vi "LinkedServer.vi"() -> ()   [LabVIEW 2012]
uses:
  <vilib>/addons/database/Auxilliary.llb/DB Tools Cursor Type.ctl
  <vilib>/addons/database/Connection.llb/DB Tools Open Connec (Path).vi
  <vilib>/addons/database/Connection.llb/Conn Execute.vi
  <vilib>/addons/database/Recordset.llb/Rec Fetch Recordset Data (R).vi
  <vilib>/addons/database/Recordset.llb/Rec Destroy - Connection.vi
  <vilib>/addons/database/NI_Database_API.lvlib
panel:
  out "recordset data":variant[][](array[variant])
  out "error out":errorcluster
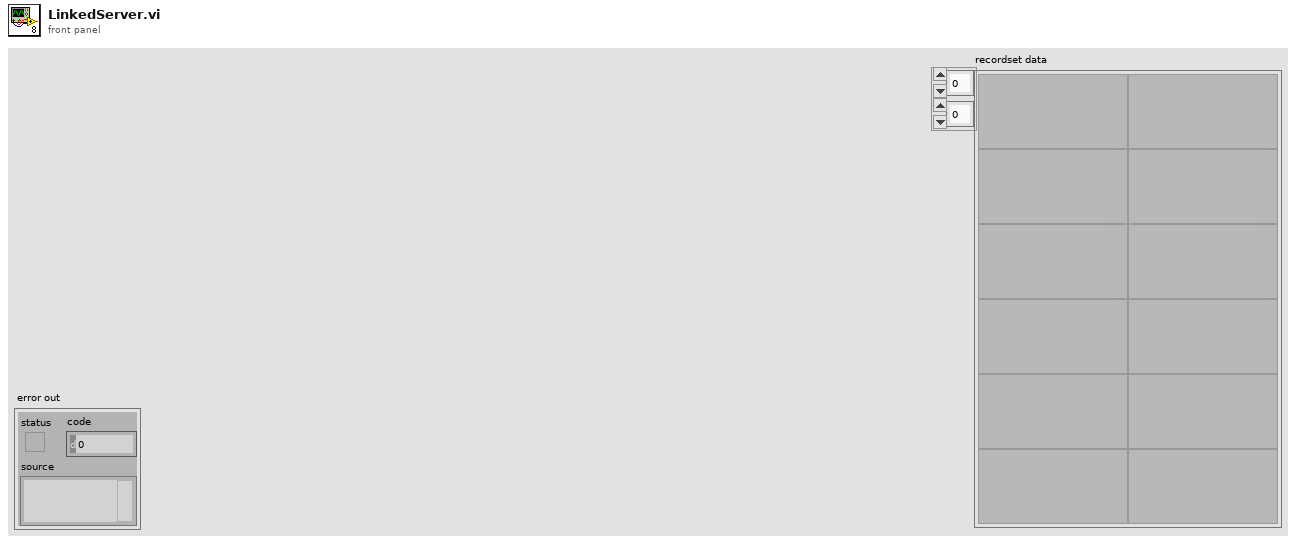
[diagram p1: front panel]
types:
  T1 = typedef "NI_Database_API.lvlib/DB Tools Cursor Type.ctl" = enum16{"forward-only", "keyset", "dynamic", "static"}
  T2 = typedef "NI_Database_API.lvlib/Conn ObjectReference.ctl" = refnum<k1>
  T3 = typedef "NI_Database_API.lvlib/Rec ObjectReference.ctl" = refnum<k1>
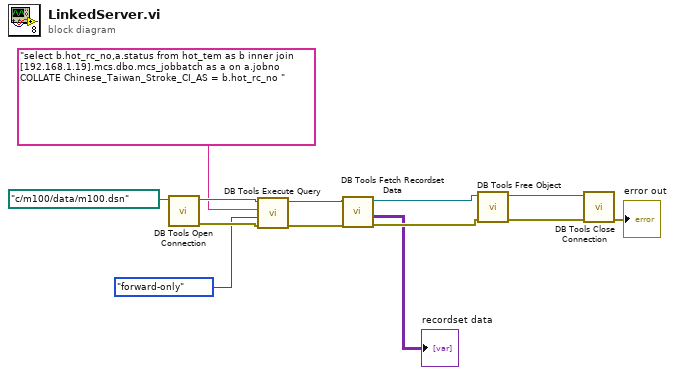
[diagram p0: block diagram]
diagram:
  n1 = call-poly <vilib>:"DB Tools Open Connection.vi"("connection information"=path "c:/m100/data/m100.dsn") -> ("error out"=w4:errorcluster, "connection reference"=w5:T2)  [unwired: 7 in]
  n2 = call-poly <vilib>:"DB Tools Execute Query.vi"("error in (no error)"=w4, "cursor type"=DB_Tools_Cursor_Type."forward-only", "SQL query"="select b.hot_rc_no,a.status from hot_tem as b inner join [192.168.1.19].mcs.dbo.mcs_jobbatch as a on a.jobno COLLATE Chinese_Taiwan_Stroke_CI_AS = b.hot_rc_no ", "connection reference"=w5) -> ("error out"=w6:errorcluster, "recordset reference"=w7:T3)  [unwired: 4 in]
  n3 = call-poly <vilib>:"DB Tools Fetch Recordset Data.vi"("error in (no error)"=w6, "recordset reference"=w7) -> ("error out"=w8:errorcluster, "recordset data"=→"recordset data":variant[][], "recordset reference out"=w9:T3)  [unwired: 3 in]
  n4 = call-poly <vilib>:"DB Tools Free Object.vi"("error in (no error)"=w8, "recordset reference"=w9) -> ("error out"=w10:errorcluster, "connection reference"=w11:T2)  [unwired: 8 in]
  n5 = call <vilib>:"DB Tools Close Connection.vi"("error in (no error)"=w10, "connection reference"=w11) -> ("error out"=→"error out":errorcluster)  [unwired: 5 in]
